vi "Initialize Results Array.vi"(9 "Stop Step":i32, 10 "Start Step":i32, 11 "Step Count":i32) -> (3 "Results":T1[](array[typedef]))   [LabVIEW 2020, in "MacroAssert.lvlib"]
doc: "Initializes an array of results based on the inputs."
uses:
  MacroAssert.lvlib
  CTLs/Result.ctl
  CTLs/Outcome.ctl
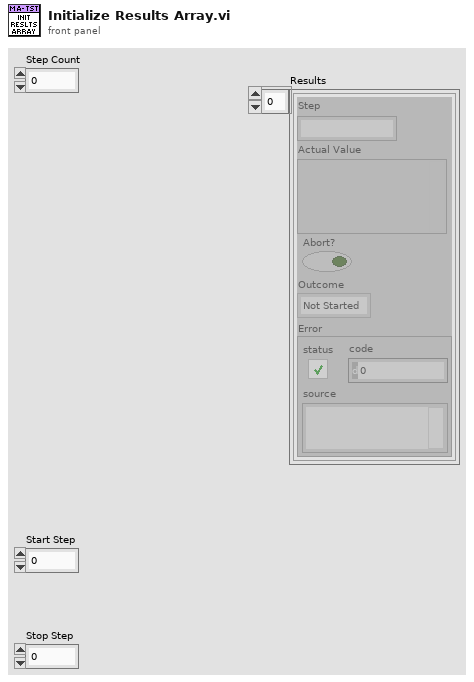
[diagram p1: front panel]
types:
  T1 = typedef "MacroAssert.lvlib/Result.ctl" = cluster{"Step":string, "Actual Value":variant, "Abort?":bool, "Outcome":T2, "Error":errorcluster}
  T2 = typedef "MacroAssert.lvlib/Outcome.ctl" = enum16{"Not Started", "Skipped", "Pass", "Fail", "Complete", "Error", "Auto Abort", "User Abort"}
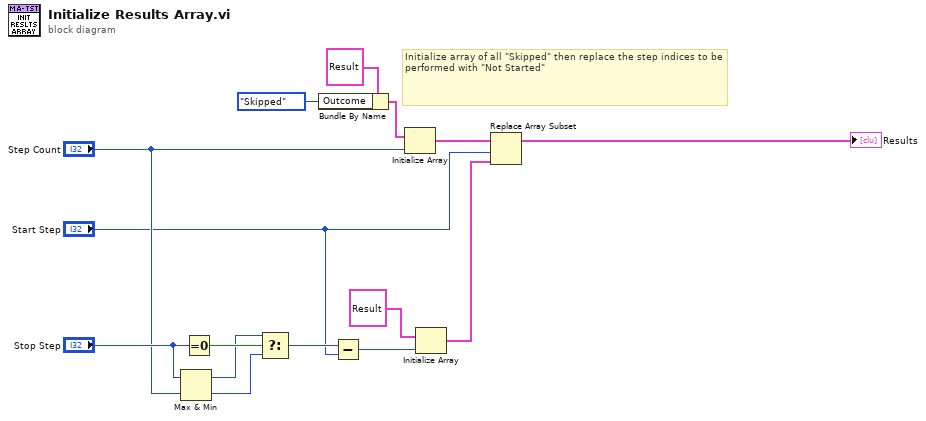
[diagram p0: block diagram]
diagram:
  # "Initialize array of all \"Skipped\" then replace the step indices to be performed with \"Not Started\""
  n1 = Max & Min(x="Stop Step", y="Step Count") -> (max(x,y)=w13:i32, min(x,y)=w14:i32)
  n2 = Equal To 0?(x="Stop Step") -> (x = 0?=w15:bool)
  n3 = Select(t=w13, s=w15, f=w14) -> (s? t:f=w8:i32)
  n4 = Bundle By Name(cluster=T1 {"Step"="", "Actual Value"=variant, "Abort?"=FALSE, "Outcome"=enum."Not Started", "Error"={"status"=FALSE, "code"=0, "source"=""}} ("Result"), "Outcome"=Outcome."Skipped" ("Result")) -> (w1:T1)
  n5 = Subtract(x=w8, y="Start Step") -> (x-y=w4:i32)
  n6 = Initialize Array(w1, "Step Count") -> (w9:T1[])
  n7 = Initialize Array(T1 {"Step"="", "Actual Value"=variant, "Abort?"=FALSE, "Outcome"=enum."Not Started", "Error"={"status"=FALSE, "code"=0, "source"=""}} ("Result"), w4) -> (w3:T1[])
  n8 = Replace Array Subset(array=w9, new element=w3, index="Start Step") -> (→"Results":T1[])
